vi "UpdateSystemHealth.vi"(7 "Qbus in":refnum<class "Qbus.lvclass">, 8 "error in (no error)":errorcluster, 9 "fpga reference":refnum<k20>, 10 "system tags":T4[](array[typedef]), 11 "system resources":T1 {"CPU Loads"."ISR (%)" format="%#.2f"; "CPU Loads"."Idle (%)" format="%#.2f"; "CPU Loads"."Background (%)" format="%#.2f"; "CPU Loads"."Normal (%)" format="%#.2f"; "CPU Loads"."Above Normal (%)" format="%#.2f"; "CPU Loads"."High (%)" format="%#.2g"; "CPU Loads"."Timed Structures (%)" format="%#.2g"; "CPU Loads"."Time Critical (%)" format="%#.2g"; "CPU Loads"."Total (%)" format="%#.2g"}) -> (0 "error out":errorcluster)   [LabVIEW 2017, in "DeviceHealth.lvlib"]
uses:
  <vilib>/addons/InsightCM/Devices/Shared/Common/DeviceHealth/DeviceHealth.lvlib
  <vilib>/addons/InsightCM/Devices/Shared/Common/DeviceHealth/controls/deviceHealthTag.ctl
  <vilib>/addons/InsightCM/Devices/Shared/Common/DeviceHealth/controls/SystemHealthTagEnum.ctl
  <vilib>/addons/InsightCM/MessageBus/Base/controls/Tag.ctl
  <vilib>/addons/InsightCM/MessageBus/Base/controls/KeyValuePair.ctl
  <vilib>/addons/SystemInfoProcess/controls/SystemResources.ctl
  <vilib>/addons/SystemInfoProcess/controls/Utilization.ctl
  <vilib>/addons/SystemInfoProcess/controls/CPULoad.ctl
  <vilib>/addons/Qbus/Qbus.lvclass
  <vilib>/addons/InsightCM/MessageBus/Base/controls/TagValueUpdate.ctl
  <vilib>/addons/InsightCM/MessageBus/Base/controls/TsTagValueString.ctl
  <vilib>/addons/InsightCM/MessageBus/Base/controls/TagValueDouble.ctl
  <vilib>/addons/InsightCM/MessageBus/Base/controls/TsTagValueDouble.ctl
  <vilib>/addons/InsightCM/MessageBus/MessageLibrary/Tag/controls/TagUpdateTagValuesRoutedMessageBody.ctl
  <vilib>/addons/InsightCM/MessageBus/MessageLibrary/Tag/controls/TagUpdateDoubleValuesRoutedMessageBody.ctl
  <vilib>/addons/InsightCM/Devices/Shared/Common/ServerComm/ServerComm.lvlib
  <vilib>/addons/SystemInfoProcess/SystemInfoProcess.lvlib
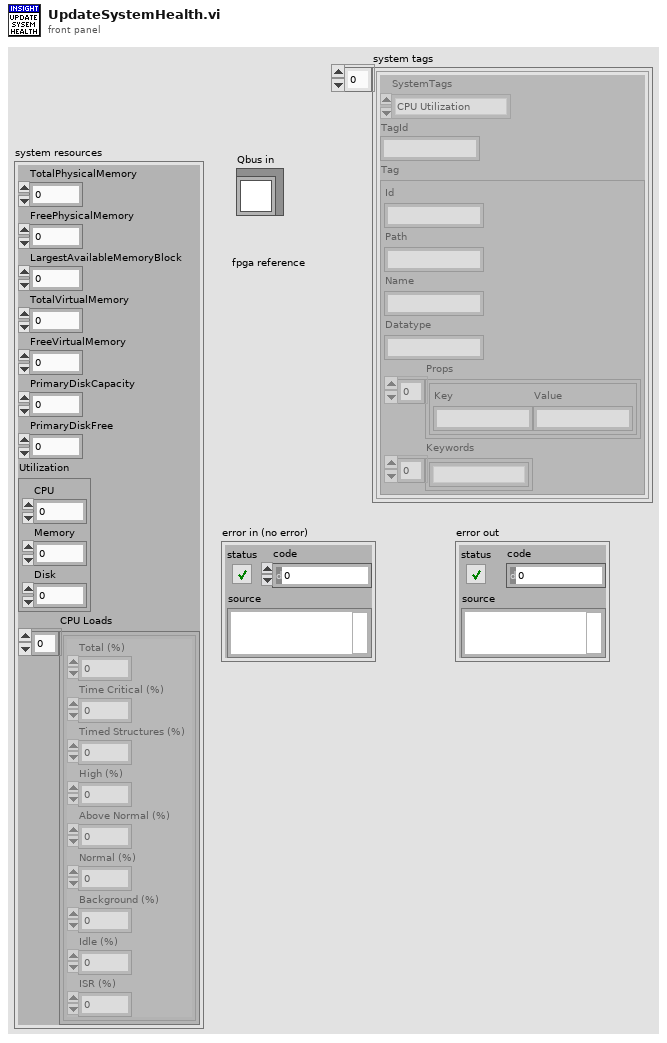
[diagram p1: front panel]
types:
  T1 = typedef "SystemInfoProcess.lvlib/SystemResources.ctl" = cluster{"TotalPhysicalMemory":dbl, "FreePhysicalMemory":dbl, "LargestAvailableMemoryBlock":dbl, "TotalVirtualMemory":dbl, "FreeVirtualMemory":dbl, "PrimaryDiskCapacity":dbl, "PrimaryDiskFree":dbl, "Utilization":T2, "CPU Loads":T3[]}
  T2 = typedef "SystemInfoProcess.lvlib/Utilization.ctl" = cluster{"CPU":dbl, "Memory":dbl, "Disk":dbl}
  T3 = typedef "SystemInfoProcess.lvlib/CPULoad.ctl" = cluster{"Total (%)":dbl, "Time Critical (%)":dbl, "Timed Structures (%)":dbl, "High (%)":dbl, "Above Normal (%)":dbl, "Normal (%)":dbl, "Background (%)":dbl, "Idle (%)":dbl, "ISR (%)":dbl}
  T4 = typedef "DeviceHealth.lvlib/deviceHealthTag.ctl" = cluster{"SystemTags":T5, "TagId":string, "Tag":T6}
  T5 = typedef "DeviceHealth.lvlib/SystemHealthTagEnum.ctl" = enum16{"CPU Utilization", "Memory Utilization", "Disk Utilization", "Total Physical Memory", "Primary Disk Free", "Chassis Temperature", "LowRateCount"}
  T6 = typedef "Tag.ctl" = cluster{"Id":string, "Path":string, "Name":string, "Datatype":string, "Props":T7[], "Keywords":string[]}
  T7 = typedef "KeyValuePair.ctl" = cluster{"Key":string, "Value":string}
  T8 = typedef "TagValueDouble.ctl" = cluster{"TagId":string, "TsValue":T9}
  T9 = typedef "TsTagValueDouble.ctl" = cluster{"Value":dbl, "Timestamp":i64}
  T10 = typedef "TagValueUpdate.ctl" = cluster{"Tag":T6, "TsValue":T11}
  T11 = typedef "TsTagValueString.ctl" = cluster{"Value":string, "Timestamp":i64}
  T12 = typedef "TagUpdateTagValuesRoutedMessageBody.ctl" = cluster{"TagsValue":T10[]}
  T13 = typedef "Message.ctl" = cluster{"Header":T14, "Body":u8[]}
  T14 = typedef "MessageHeader.ctl" = cluster{"MessageName":string, "Timestamp":i64, "CorrelationId":string, "ContentType":string, "RoutingKey":string, "Properties":T7[]}
  T15 = typedef "TagUpdateDoubleValuesRoutedMessageBody.ctl" = cluster{"TagsValue":T8[]}
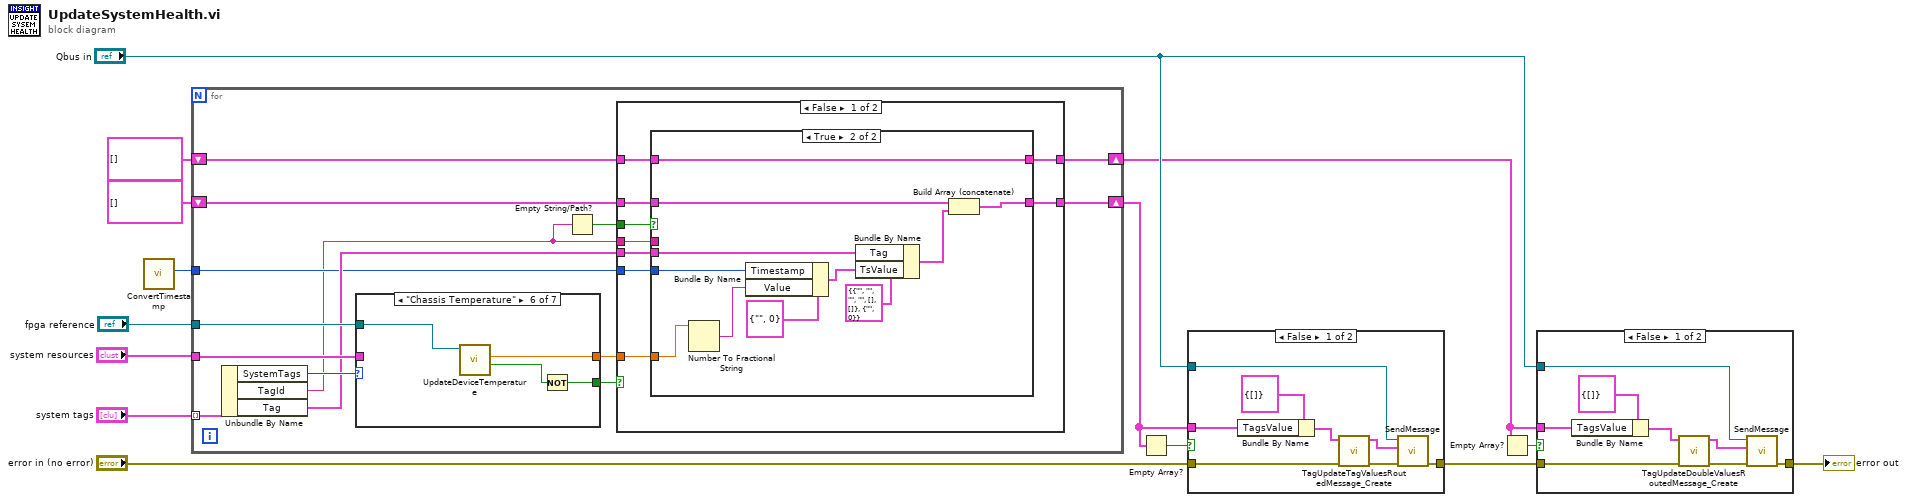
[diagram p0: block diagram]
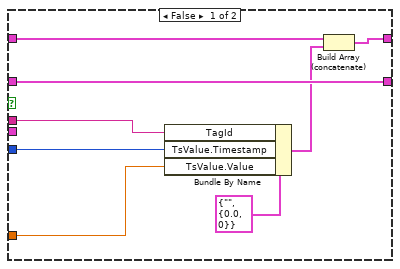
[diagram p4: hidden frame]
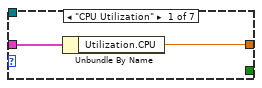
[diagram p6: hidden frame]
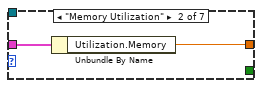
[diagram p7: hidden frame]
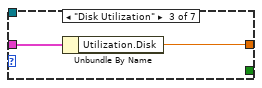
[diagram p8: hidden frame]
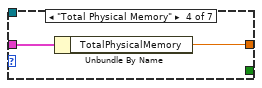
[diagram p9: hidden frame]
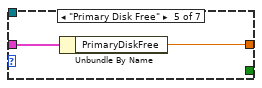
[diagram p10: hidden frame]
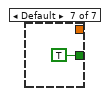
[diagram p11: hidden frame]
diagram:
  n1 = call <vilib>:"ConvertTimestamp.vi"() -> ("Timestamp out"=w11:i64)  [unwired: 11 in]
  n2 = for {
    tunnel: "system tags" -> [w26] mode=indexing
    tunnel: "system resources" -> [w28]
    tunnel: "fpga reference" -> [w25]
    shift-right: [w16] -> w2
    shift-left: T8[] [] -> [w15]
    shift-right: [w19] -> w7
    shift-left: T10[] [] -> [w18]
    tunnel: w11 -> [w20]
    n3 = Unbundle By Name(w26) -> ("SystemTags"=w27:T5, "TagId"=w17:string, "Tag"=w22:T6)
    n4 = case shown="\"Chassis Temperature\"" w27 {
      tunnel: w28 -> [w60 w62 w64 w66 w68 _ _]
      tunnel: [w59 w61 w63 w65 w67 w71 _] -> w21
      tunnel: w25 -> [_ _ _ _ _ w72 _]
      tunnel: [_ _ _ _ _ w69 TRUE] -> w24
      frame "CPU Utilization" {
        n5 = Unbundle By Name(w60) -> ("Utilization.CPU"=w59:dbl)
      }
      frame "Memory Utilization" {
        n6 = Unbundle By Name(w62) -> ("Utilization.Memory"=w61:dbl)
      }
      frame "Disk Utilization" {
        n7 = Unbundle By Name(w64) -> ("Utilization.Disk"=w63:dbl)
      }
      frame "Total Physical Memory" {
        n8 = Unbundle By Name(w66) -> ("TotalPhysicalMemory"=w65:dbl)
      }
      frame "Primary Disk Free" {
        n9 = Unbundle By Name(w68) -> ("PrimaryDiskFree"=w67:dbl)
      }
      frame "Chassis Temperature" {
        n10 = call <vilib>:"UpdateDeviceTemperature.vi"("fpga reference"=w72) -> ("valid"=w70:bool, "temperature"=w71:dbl)  [unwired: 8 in, 1 out]
        n11 = Not(x=w70) -> (.not. x?=w69:bool)
      }
      frame Default {
      }
    }
    n12 = Empty String/Path?(string/path=w17) -> (empty?=w23:bool)
    n13 = case shown="False" w24 {
      tunnel: w23 -> [w37 _]
      tunnel: w22 -> [w36 _]
      tunnel: w21 -> [w35 _]
      tunnel: w20 -> [w34 _]
      tunnel: [w33 w58] -> w19
      tunnel: w18 -> [w32 w58]
      tunnel: w17 -> [w31 _]
      tunnel: [w30 w57] -> w16
      tunnel: w15 -> [w29 w57]
      frame False {
        n14 = case shown="True" w37 {
          tunnel: w36 -> [_ w50]
          tunnel: w35 -> [w41 w54]
          tunnel: w34 -> [w44 w52]
          tunnel: [w45 w48] -> w33
          tunnel: w32 -> [w45 w47]
          tunnel: w31 -> [w43 _]
          tunnel: [w39 w46] -> w30
          tunnel: w29 -> [w38 w46]
          frame False {
            n15 = Bundle By Name(cluster=T8 {"TagId"="", "TsValue"={"Value"=0.0, "Timestamp"=0}} ("TagValue"), "TagId"=w43, "TsValue.Timestamp"=w44, "TsValue.Value"=w41) -> (w40:T8)
            n16 = Build Array (concatenate)(w38, w40) -> (w39:T8[])
          }
          frame True {
            n17 = Number To Fractional String(number=w54) -> (F-format string=w53:string)  [unwired: 3 in]
            n18 = Bundle By Name(cluster=T11 {"Value"="", "Timestamp"=0} ("TsValue"), "Timestamp"=w52, "Value"=w53) -> (w51:T11)
            n19 = Bundle By Name(cluster=T10 {"Tag"={"Id"="", "Path"="", "Name"="", "Datatype"="", "Props"=[], "Keywords"=[]}, "TsValue"={"Value"="", "Timestamp"=0}} ("TagValue"), "Tag"=w50, "TsValue"=w51) -> (w49:T10)
            n20 = Build Array (concatenate)(w47, w49) -> (w48:T10[])
          }
        }
      }
      frame True {
      }
    }
  }
  n21 = Empty Array?(array=w7) -> (empty?=w9:bool)
  n22 = case shown="False" w9 {
    tunnel: "error in (no error)" -> [w77 w82]
    tunnel: [w81 w82] -> w5
    tunnel: w7 -> [w78 _]
    tunnel: "Qbus in" -> [w80 _]
    frame False {
      n23 = Bundle By Name(cluster=T12 {"TagsValue"=[]} ("TagUpdateTagValuesRoutedMessage"), "TagsValue"=w78) -> (w75:T12)
      n24 = call <vilib>:"TagUpdateTagValuesRoutedMessage_Create.vi"("error in (no error)"=w77, "TagUpdateTagValuesRoutedMessage"=w75) -> ("error out"=w76:errorcluster, "Message"=w74:T13)  [unwired: 8 in]
      n25 = call <vilib>:"SendMessage.vi"("error in (no error)"=w76, "message"=w74, "Qbus in"=w80) -> ("error out"=w81:errorcluster)  [unwired: 7 in, 1 out]
    }
    frame True {
    }
  }
  n26 = Empty Array?(array=w2) -> (empty?=w6:bool)
  n27 = case shown="False" w6 {
    tunnel: w5 -> [w88 w91]
    tunnel: [w90 w91] -> w1
    tunnel: w2 -> [w83 _]
    tunnel: "Qbus in" -> [w89 _]
    frame False {
      n28 = Bundle By Name(cluster=T15 {"TagsValue"=[]} ("Body"), "TagsValue"=w83) -> (w85:T15)
      n29 = call <vilib>:"TagUpdateDoubleValuesRoutedMessage_Create.vi"("error in (no error)"=w88, "TagUpdateDoubleValuesRoutedMessage"=w85) -> ("error out"=w87:errorcluster, "Message"=w84:T13)  [unwired: 8 in]
      n30 = call <vilib>:"SendMessage.vi"("error in (no error)"=w87, "message"=w84, "Qbus in"=w89) -> ("error out"=w90:errorcluster)  [unwired: 7 in, 1 out]
    }
    frame True {
    }
  }
  "error out" <- w1
